vi "readFromXML.vi"(8 "error in (no error)":errorcluster, 10 "XML in":string="<MccAzElTrack>\n<mccTrack>Off</mccTrack>\n</MccAzElTrack>", 11 "MccAzElTrack in":refnum<class "MccAzElTrack.lvclass">) -> (0 "error out":errorcluster={"status"=TRUE, "code"=1, "source"="(Unknown Enum Value <Op>) Set Enum String Value__ogtk.vi in 686C45C435F7D6D638AFE3BF1019BA0E->A5AE8EA5BC9E882D19C00E2FAEC17B15:1->Easy Parse XML__JKI EasyXML.vi->MccAzElTrack.lvclass:readFromXML.vi\r\n"}, 3 "MccAzElTrack out":refnum<class "MccAzElTrack.lvclass">)   [LabVIEW 2022 SP3, in "TCSDataDefinitions.lvlib" / "TCSMountControlCommand.lvlib" / "CommandsForAzElAxes.lvlib" / "MccAzElTrack.lvclass"]
uses:
  MccAzElTrack.lvclass
  Enumerations/MountTrackStates.ctl
  MccAzElTrack.lvclass/MccAzElTrack.ctl
  CommandsForAzElAxes.lvclass
  <userlib>/Common/XML/XMLParser/XMLParser.lvclass
  TCSMountControlCommand.lvlib
panel:
  out "data":T1
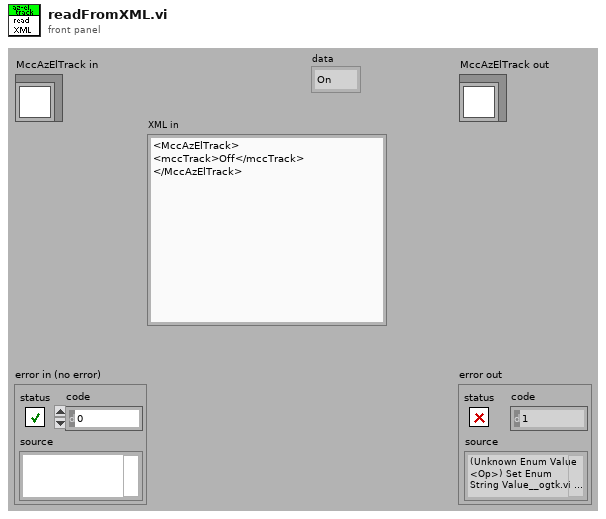
[diagram p1: front panel]
types:
  T1 = typedef "TCSDataDefinitions.lvlib/TCSMountControlCommand.lvlib/MountTrackStates.ctl" = enum16{"On", "Off"}
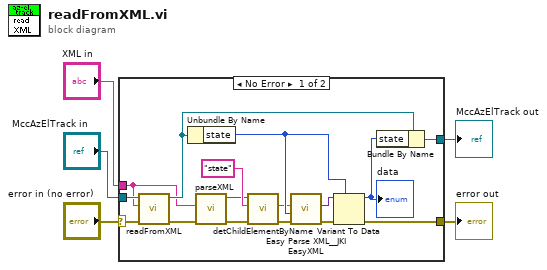
[diagram p0: block diagram]
diagram:
  n1 = case shown="No Error" "error in (no error)" {
    selector: "error in (no error)" -> [w20 w23]
    tunnel: [w13 w23] -> w4
    tunnel: [w14 w22] -> w2
    tunnel: "MccAzElTrack in" -> [w21 w22]
    tunnel: "XML in" -> [w12 _]
    frame No Error {
      n2 = call-parent "readFromXML.vi"("error in (no error)"=w20, "XML in"=w12, "CommandsForAzElAxes in"=w21) -> ("error out"=w9:errorcluster, "CommandsForAzElAxes out"=w15:refnum<class "MccAzElTrack.lvclass">)  [unwired: 7 out]
      n3 = Unbundle By Name(w15) -> ("state"=w19:T1)
      n4 = call <userlib>:"parseXML.vi"("error in (no error)"=w9, "XMLString in"=w12) -> ("error out"=w8:errorcluster, "Element out"=w6:refnum<class "XMLParser.lvclass">)  [unwired: 8 in]
      n5 = call <userlib>:"detChildElementByName.vi"("error in (no error)"=w8, "childName"="state" ("ChildName"), "Element in"=w6) -> ("error out"=w7:errorcluster, "childXML"=w10:string)  [unwired: 5 in, 2 out]
      n6 = call <vilib>:"Easy Parse XML__JKI EasyXML.vi"("error in (no error)"=w7, "LabVIEW Data (Type)"=w19, "XML String"=w10) -> ("error out"=w17:errorcluster, "LabVIEW Data"=w18:variant)  [unwired: 7 out]
      n7 = Variant To Data(error in=w17, type=w19, Variant=w18) -> (data=w16:T1, error out=w13:errorcluster)
      "data" <- w16
      n8 = Bundle By Name(cluster=w15, "state"=w16) -> (w14:refnum<class "MccAzElTrack.lvclass">)
    }
    frame Error {
    }
  }
  "error out" <- w4
  "MccAzElTrack out" <- w2
